vi "Scout.vi"() -> ()   [LabVIEW 2013]
panel:
  in  "What Can They Do in Teleop?":string
  in  "How Does it Work?":string
  in  "Autonomous?":string(combo)="Other"
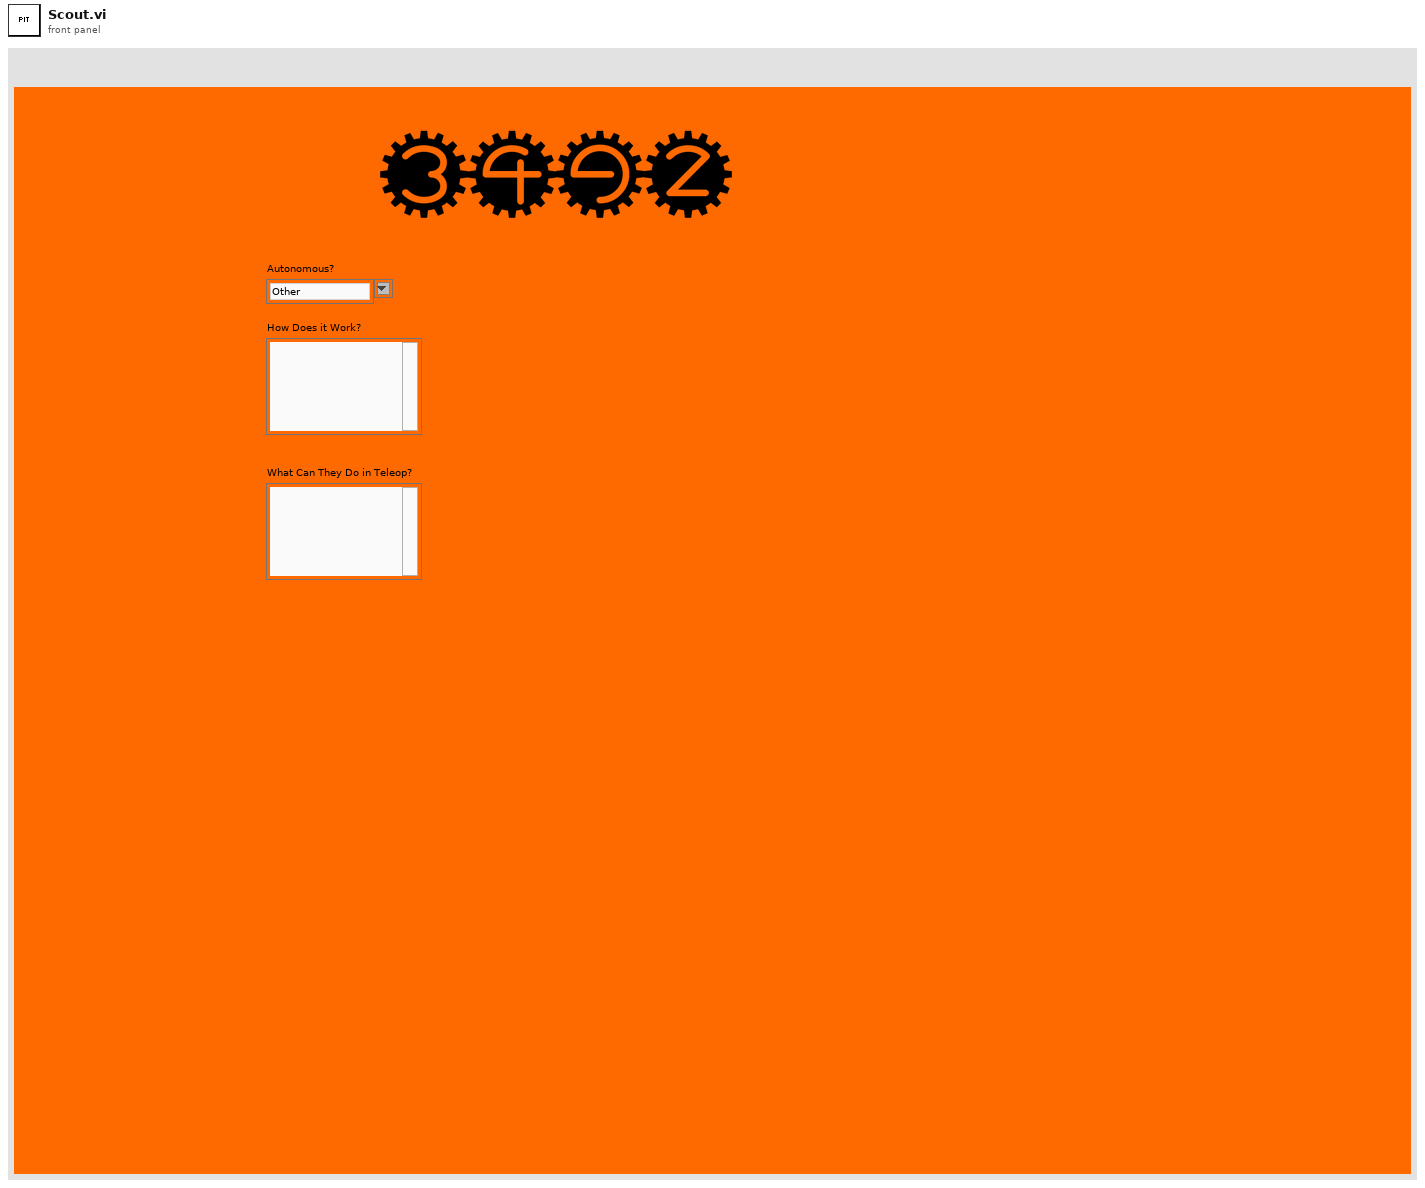
[diagram p1: front panel]
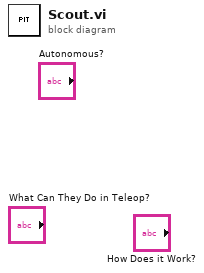
[diagram p0: block diagram]
diagram:
